vi "User Selection.vi"(2 "error in (no error)":errorcluster, 3 "Cluster":T2, 4 "file path (use dialog)":path) -> (0 "error out":errorcluster, 1 "Cluster 2":T1)   [LabVIEW 2017]
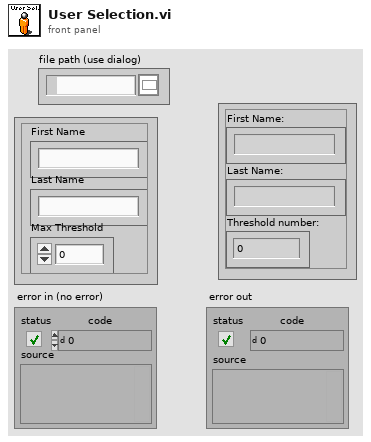
[diagram p1: front panel]
types:
  T1 = cluster{"First Name:":string, "Last Name:":string, "Threshold number:":dbl}
  T2 = cluster{"First Name":string, "Last Name":string, "Max Threshold":dbl}
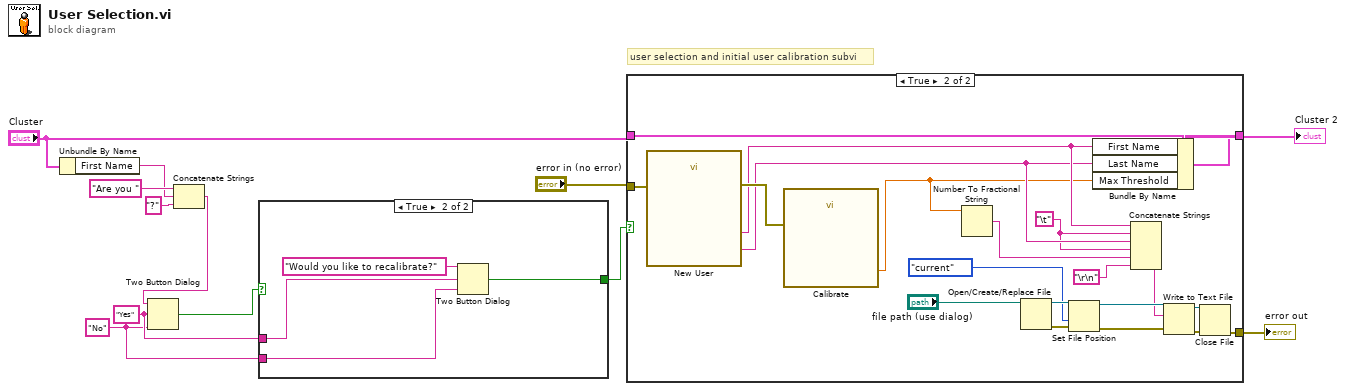
[diagram p0: block diagram]
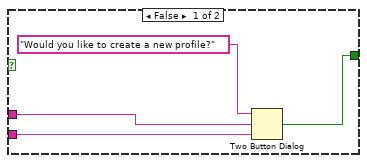
[diagram p2: hidden frame]
diagram:
  w4 = "No" ("F button name (\"Cancel\")")
  w5 = "Yes" ("T button name (\"OK\")")
  # "user selection and initial user calibration subvi"
  n1 = Unbundle By Name("Cluster") -> ("First Name"=w9:string)
  n2 = Concatenate Strings("Are you " ("string"), w9, "?" ("string")) -> (w7:string)
  n3 = Two Button Dialog(message=w7, 1:w4, 2:w5) -> (T button?=w2:bool)
  n4 = case shown="True" w2 {
    tunnel: w5 -> [w15 w19]
    tunnel: w4 -> [w14 w18]
    tunnel: [w13 w17] -> w3
    frame False {
      n5 = Two Button Dialog(message="Would you like to create a new profile?", 1:w14, 2:w15) -> (T button?=w13:bool)
    }
    frame True {
      n6 = Two Button Dialog(message="Would you like to recalibrate?", 1:w18, 2:w19) -> (T button?=w17:bool)
    }
  }
  n7 = case shown="True" w3 {
    tunnel: "Cluster" -> [w22 w42]
    tunnel: [w22 w41] -> w12
    tunnel: "error in (no error)" -> [w21 w40]
    tunnel: [w21 w23] -> w1
    frame False {
    }
    frame True {
      w27 = "\t"
      n8 = call "New User"("error in (no error)"=w40) -> ("Last Name:"=w31:string, "First Name:"=w32:string, "error out"=w39:errorcluster)  [unwired: 15 in, 1 out]
      n9 = call "Calibrate"("error in (no error)"=w39) -> ("Calibration Value:"=w30:dbl)  [unwired: 16 in, 2 out]
      n10 = Number To Fractional String(number=w30) -> (F-format string=w29:string)  [unwired: 3 in]
      n11 = Open/Create/Replace File(file path (use dialog)="file path (use dialog)") -> (refnum out=w35:refnum<file>, error out=w34:errorcluster)  [unwired: 5 in, 1 out]
      n12 = Set File Position(refnum=w35, from (0:start)=enum16{"start", "end", "current"}."current", error in=w34) -> (refnum out=w37:refnum<file>, error out=w38:errorcluster)  [unwired: 1 in]
      n13 = Bundle By Name(cluster=w42, "First Name"=w32, "Last Name"=w31, "Max Threshold"=w30) -> (w41:T2)
      n14 = Concatenate Strings(w32, w27, w31, w27, w29, "\r\n") -> (w26:string)
      n15 = Write to Text File(file (use dialog)=w37, text=w26, error in=w38) -> (refnum out=w24:refnum<file>, error out=w25:errorcluster)  [unwired: 1 in, 1 out]
      n16 = Close File(refnum=w24, error in=w25) -> (error out=w23:errorcluster)  [unwired: 1 out]
    }
  }
  "error out" <- w1
  "Cluster 2" <- w12
